vi "Skywater.vi"() -> ()   [LabVIEW 2018]
uses:
  Globals.vi
  <vilib>/Utility/file.llb/Write Delimited Spreadsheet (DBL).vi
panel:
  in  "current limit range (A)":dbl=3.2e-05 format="%#_6p"
  in  "RRAM Mode":u16(ring)=1 items=["1T1R", "1T4R", "1T8R"]
  in  "Addr hold time (s)":dbl=0.001 caption="Time Target (s)" format="%#_6p"
  in  "Initial address":i32
  in  "Stride":i32=8
  in  "Final address":i32=4096
  out "Current address":i32=4096
  in  "Mode":T1(tab)=enum."Target"
  in  "FORM outfile":path=path "C:/Users/RSG/Desktop/NI-Skywater-Test-Setup/eray/1T8R_form"
  out "FORM resistance (ohm)":dbl=10056.36151540716 format="%#_6p"
  out "FORM WL voltage (V)":dbl=1.2
  out "FORM BL voltage (V)":dbl=1.0
  out "formed?":bool=TRUE
  in  "SET target resistance (ohm)":dbl format="%#_6p"
  out "SET resistance (ohm)":dbl format="%#_6p"
  out "SET WL voltage (V)":dbl
  out "SET BL voltage (V)":dbl
  out "set?":bool
  in  "SET outfile":path=path "C:/Users/RSG/Desktop/NI-Skywater-Test-Setup/set.csv"
  in  "RESET target resistance (ohm)":dbl=50000.0 format="%#_6p"
  in  "RESET outfile":path=path "C:/Users/RSG/Desktop/NI-Skywater-Test-Setup/prereset.csv"
  out "reset?":bool=TRUE
  out "RESET SL voltage (V)":dbl=0.1
  out "RESET WL voltage (V)":dbl=0.1
  out "RESET resistance (ohm)":dbl=-27076590.237838075 format="%#_6p"
  in  "aperture time (s)":dbl=0.0005 format="%#_6p"
  in  "channel list":string="BL_SEL_0"
  in  "voltage level (V)":dbl=0.2 format="%#_6p"
  in  "settling time (s)":dbl=0.001 caption="Time Target (s)" format="%#_6p"
  out "currents (A)":dbl[][](array[numeric])=[[2.5991655032025314e-06], [2.6178851900457248e-06], [2.629369660501652e-06], [2.5730383329152406e-06], [2.541800573275067e-06], [2.630403262842684e-06], [2.5273875628528547e-06], [2.615186339488569e-06], [2.5948014044292527e-06], [2.4742144646418167e-06], [2.5204394582269958e-06], [2.4999971008154232e-06], [2.519922657056459e-06], [2.621330531182484e-06], [2.4824832833700937e-06], [2.4807606128016933e-06], [2.5330149533762534e-06], [2.6165644759432856e-06], [2.6238571146828077e-06], [2.569765258835313e-06], [2.5066006713275767e-06], [2.577459854040776e-06], [2.469792943516261e-06], [2.4861583139160038e-06], [2.607147210169401e-06], [2.5890591692012994e-06], [2.474673843460035e-06], [2.5888294797921905e-06], [2.6161050971250466e-06], [2.507749118373163e-06], [2.542030262684197e-06], [2.56959299177846e-06], [2.56224293068664e-06], [2.578608301086383e-06], [2.471630458789216e-06], [2.5237125323069446e-06], [2.5285934322507392e-06], [2.587336498632878e-06], [2.482311016313262e-06], [2.568214855323765e-06], [2.6001416831912863e-06], [2.592906466804041e-06], [2.4948865114625405e-06], [2.5907244174174017e-06], [2.5169366947379384e-06], [2.483287196301996e-06], [2.56482693653922e-06], [2.5010881255087116e-06], [2.5543186460720477e-06], [2.615817985363661e-06], [2.619837550023234e-06], [2.523310575841004e-06], [2.559946036595467e-06], [2.472491794073395e-06], [2.581594263404925e-06], [2.477085582255804e-06], [2.5706265941195135e-06], [2.4692187199934886e-06], [2.4722621046643074e-06], [2.48948881034823e-06], [2.573497711733479e-06], [2.603759291384898e-06], [2.5118261053850556e-06], [2.5823407539845498e-06], [2.503844398418165e-06], [2.6069749431125487e-06], [2.538872033308824e-06], [2.489718499757339e-06], [2.4820813269041528e-06], [2.5377235862631957e-06], [2.57389966819942e-06], [2.5408243932863126e-06], [2.531694239273856e-06], [2.5649417812437956e-06], [2.5744164693699567e-06], [2.5070600501458364e-06], [2.4714007693800864e-06], [2.5745887364268094e-06], [2.5535147331401244e-06], [2.5427193309115445e-06], [2.5436380885480013e-06], [2.568214855323765e-06], [2.6206988853074342e-06], [2.5368048286267393e-06], [2.5548354472425636e-06], [2.6078937007490262e-06], [2.56333395537997e-06], [2.6108222407152904e-06], [2.618861370034479e-06], [2.551504950810338e-06], [2.577804388154481e-06], [2.516190204158293e-06], [2.4707691235050155e-06], [2.631207175774628e-06], [2.567468364744098e-06], [2.481736792790448e-06], [2.624948139376138e-06], [2.6001991055435636e-06], [2.6293122381493748e-06], [2.6262688534785556e-06], [2.621387953534782e-06], [2.6042186702031576e-06], [2.6057116513624076e-06], [2.6274747228764197e-06], [2.5883126786216535e-06], [2.5067155160321314e-06], [2.6222492888189616e-06], [2.485641512745488e-06], [2.517855452374416e-06], [2.6282212134560864e-06], [2.6235700029214215e-06], [2.5512178390489516e-06], [2.56224293068664e-06], [2.4763965140284565e-06], [2.6070323654648468e-06], [2.5409966603431653e-06], [2.473295707005339e-06], [2.5963518079408215e-06], [2.4696780988116856e-06], [2.5257223146367313e-06], [2.497700206724229e-06], [2.5825704433937e-06], [2.5093569442370093e-06], [2.618000034750258e-06], [2.5005139019859395e-06], [2.553916689606086e-06], [2.5049354231114744e-06], [2.623971959387404e-06], [2.618000034750258e-06], [2.505969025452506e-06], [2.5621855083343838e-06], [2.5615538624593132e-06], [2.629139971092564e-06], [2.63137944283146e-06], [2.5304883698759716e-06], [2.482253593960964e-06], [2.5134913536011584e-06], [2.512974552430642e-06], [2.4726066387779705e-06], [2.5681574329714667e-06], [2.607262054873977e-06], [2.543810355604854e-06], [2.5335891768990678e-06], [2.575335227006434e-06], [2.625752052308061e-06], [2.5207265699883824e-06], [2.481564525733637e-06], [2.5329575310239765e-06], [2.482311016313262e-06], [2.599854571429879e-06], [2.5806180834161697e-06], [2.6027831113961435e-06], [2.625005561728436e-06], [2.5987061243842925e-06], [2.5584530554362175e-06], [2.544556846184479e-06], [2.5993951926116403e-06], [2.5287082769552935e-06], [2.6237996923305516e-06], [2.5749906928927503e-06], [2.509242099532476e-06], [2.532096195739776e-06], [2.573612556438034e-06], [2.5942271809064803e-06], [2.6215027982393368e-06], [2.470654278800461e-06], [2.6146695383180532e-06], [2.510447968930319e-06], [2.4926470397236026e-06], [2.5546057578334547e-06], [2.59313615621315e-06], [2.616162519477324e-06], [2.604850316078228e-06], [2.517453495908475e-06], [2.6008307514186338e-06], [2.589920504485479e-06], [2.5769430528702803e-06], [2.578608301086383e-06], [2.5006287466904938e-06], [2.5325555745580356e-06], [2.562013241277531e-06], [2.563276533027693e-06], [2.561496440107015e-06], [2.5335891768990678e-06], [2.6061710301806466e-06], [2.6077214336922154e-06], [2.5973854102818537e-06], [2.5887720574398924e-06], [2.535771226285707e-06], [2.6041612478508595e-06], [2.625177828785226e-06], [2.5608073718796465e-06], [2.6279341016946795e-06], [2.6260391640694467e-06], [2.6308052193086663e-06], [2.567640631800951e-06], [2.607836278396749e-06], [2.6220195994098734e-06], [2.6283360581606407e-06], [2.5542612237197704e-06], [2.6263836981831314e-06], [2.4892016985868226e-06], [2.603185067862126e-06], [2.5605202601182815e-06], [2.5732680223243495e-06], [2.5300864134099892e-06], [2.6169090100569907e-06], [2.4893739656436753e-06], [2.4796121657560857e-06], [2.5791825246091555e-06], [2.6038741360894526e-06], [2.5487486779009052e-06], [2.4730660175962303e-06], [2.497700206724229e-06], [2.5769430528702803e-06], [2.5582807883793648e-06], [2.5942846032587576e-06], [2.5919877091675636e-06], [2.545360759116402e-06], [2.5386997662519713e-06], [2.5909541068265106e-06], [2.5470260073325256e-06], [2.566032805937126e-06], [2.5914134856447708e-06], [2.583087244564216e-06], [2.5805032387116155e-06], [2.5981319008614785e-06], [2.4712859246755525e-06], [2.5709711282331555e-06], [2.5671812529827123e-06], [2.4912114809165884e-06], [2.5096440559984163e-06], [2.499824833758571e-06], [2.543867777957152e-06], [2.6064581419420536e-06], [2.623512580569123e-06], [2.4878809844843626e-06], [2.4827129727792026e-06], [2.5833743563255815e-06], [2.615358606545422e-06], [2.537321629797255e-06], [2.5223918182045266e-06], [2.630001306376764e-06], [2.574186779960827e-06], [2.5205543029315716e-06], [2.629943884024466e-06], [2.4911540585643323e-06], [2.6046780490213754e-06], [2.5598886142431898e-06], [2.592906466804041e-06], [2.4807031904493948e-06], [2.56959299177846e-06], [2.5762539846429117e-06], [2.5793547916660083e-06], [2.624488760557899e-06], [2.519635545295094e-06], [2.490063033871002e-06], [2.5528830872650543e-06], [2.5377810086154937e-06], [2.610477706601648e-06], [2.540135325058944e-06], [2.5798141704842676e-06], [2.475879712857919e-06], [2.584293113962059e-06], [2.625292673489801e-06], [2.6155882959545307e-06], [2.4764539363807334e-06], [2.6153011841931238e-06], [2.6170812771137803e-06], [2.554663180185711e-06], [2.544556846184479e-06], [2.54237479679784e-06], [2.601462397293725e-06], [2.580273549302486e-06], [2.4928193067804553e-06], [2.547944764969003e-06], [2.573497711733479e-06], [2.5141229994762497e-06], [2.56810001061919e-06], [2.6310923310700733e-06], [2.5039592431227196e-06], [2.5781489222681238e-06], [2.6303458404904065e-06], [2.6269004993536473e-06], [2.5631616883231175e-06], [2.5672960976872873e-06], [2.593767802088221e-06], [2.6223067111712596e-06], [2.475305489335126e-06], [2.620296928841452e-06], [2.5483467214349647e-06], [2.481909059847301e-06], [2.5135487759534145e-06], [2.5127448630214917e-06], [2.5707414388240677e-06], [2.5985338573274397e-06], [2.596926031463636e-06], [2.6220770217621507e-06], [2.5457627155823845e-06], [2.478176606949113e-06], [2.554433490776602e-06], [2.6308052193086663e-06], [2.6127171783405435e-06], [2.6221918664666842e-06], [2.473812508175855e-06], [2.6189187923867565e-06], [2.5029256407816874e-06], [2.6084679242718614e-06], [2.4769133151989516e-06], [2.6224789782280912e-06], [2.533991133365029e-06], [2.6215602205916137e-06], [2.5078065407254612e-06], [2.6166793206478403e-06], [2.5091846771801773e-06], [2.6206988853074342e-06], [2.554146379015195e-06], [2.6041038254986034e-06], [2.57522038230188e-06], [2.5267559169777634e-06], [2.599854571429879e-06], [2.6041612478508595e-06], [2.4777746504831306e-06], [2.613578513624744e-06], [2.5751055375973045e-06], [2.577746965802183e-06], [2.47369766347128e-06], [2.561726129516124e-06], [2.6300587287290415e-06], [2.5759668728815047e-06], [2.551906907276299e-06], [2.571545351755991e-06], [2.5317516616261127e-06], [2.6150140724317164e-06], [2.5413986168091058e-06], [2.617253544170633e-06], [2.5444420014799246e-06], [2.5085530313050864e-06], [2.516075359453738e-06], [2.4776598057785764e-06], [2.5530553543219066e-06], [2.607549166635384e-06], [2.606917520760292e-06], [2.608927303090079e-06], [2.6161050971250466e-06], [2.5607499495273696e-06], [2.5237699546592012e-06], [2.6057690737147057e-06], [2.625292673489801e-06], [2.563793334198188e-06], [2.4999971008154232e-06], [2.622134444114407e-06], [2.586360318644123e-06], [2.516821850033384e-06], [2.631034908717775e-06], [2.6286231699220273e-06], [2.5600034589477444e-06], [2.551906907276299e-06], [2.4902353009278548e-06], [2.4784062963582427e-06], [2.6220770217621507e-06], [2.5276746746142617e-06], [2.4739273528804097e-06], [2.6163922088864536e-06], [2.5186593653063185e-06], [2.5049354231114744e-06], [2.5821110645754197e-06], [2.6227086676372213e-06], [2.6302884181381504e-06], [2.6271876111150543e-06], [2.553399888435549e-06], [2.6008307514186338e-06], [2.615645718306829e-06], [2.614037892442962e-06], [2.4816219480858723e-06], [2.6233977358645687e-06], [2.5385849215474166e-06], [2.5449013802981635e-06], [2.606056185476071e-06], [2.6290251263879886e-06], [2.5384126544905643e-06], [2.6303458404904065e-06], [2.6101331724879637e-06], [2.622134444114407e-06], [2.623512580569123e-06], [2.6264411205353875e-06], [2.6242016487964916e-06], [2.5740145129039747e-06], [2.5626448871526016e-06], [2.597787366747815e-06], [2.600084260839009e-06], [2.4742144646418167e-06], [2.5307180592850805e-06], [2.6121429548177503e-06], [2.60525227254419e-06], [2.480530923392605e-06], [2.5884849456784855e-06], [2.6082382348627105e-06], [2.4721472599597527e-06], [2.5414560391613623e-06], [2.5475428085030415e-06], [2.61409531479526e-06], [2.510907347748578e-06], [2.4979873184856366e-06], [2.5218175946817123e-06], [2.5273875628528547e-06], [2.5907244174174017e-06], [2.6175406559320608e-06], [2.5682722776760214e-06], [2.561209328345608e-06], [2.514410111237636e-06], [2.4940251761782983e-06], [2.497298250258268e-06], [2.4703097446867977e-06], [2.5262391158072476e-06], [2.5704543270626608e-06], [2.561726129516124e-06], [2.591528330349325e-06], [2.4819664821995778e-06], [2.6217899100007645e-06], [2.5914134856447708e-06], [2.5849247598371503e-06], [2.546681473218862e-06], [2.532153618092074e-06], [2.503385019599905e-06], [2.5940549138496275e-06], [2.606917520760292e-06], [2.4925896173713464e-06], [2.56333395537997e-06], [2.483402041006571e-06], [2.573669978790332e-06], [2.6061710301806466e-06], [2.613061712454228e-06], [2.5511029943443973e-06], [2.615128917136292e-06], [2.5571897636860553e-06], [2.618976214739055e-06], [2.6184019912162406e-06], [2.6062284525329235e-06], [2.580388394007061e-06], [2.4821387492564098e-06], [2.5208414146929366e-06], [2.533474332194513e-06], [2.5848673374848734e-06], [2.513663620657969e-06], [2.4894313879959315e-06], [2.5806180834161697e-06], [2.5439252003094294e-06], [2.591011529178809e-06], [2.5729234882106656e-06], [2.4692187199934886e-06], [2.5856138280644982e-06], [2.5888869021444467e-06], [2.603529601975789e-06], [2.5286508546030166e-06], [2.4697355211639833e-06], [2.5208414146929366e-06], [2.4970111384968606e-06], [2.6300587287290415e-06], [2.6188039476822023e-06], [2.6230532017509264e-06], [2.5888869021444467e-06], [2.6261540087740225e-06], [2.5642527130164477e-06], [2.5934806903268135e-06], [2.6163922088864536e-06], [2.569765258835313e-06], [2.4956330020421652e-06], [2.5973854102818537e-06], [2.559084701311267e-06], [2.5985338573274397e-06], [2.543580666195745e-06], [2.609329259556041e-06], [2.5145823782944467e-06], [2.5898630821332227e-06], [2.5716601964605453e-06], [2.543810355604854e-06], [2.609501526612872e-06], [2.4861583139160038e-06], [2.6295993499107818e-06], [2.586130629235035e-06], [2.6282786358083426e-06], [2.4804160786880505e-06], [2.588714635087615e-06], [2.5631042659708406e-06], [2.6056542290101515e-06], [2.5608073718796465e-06], [2.4733531293576372e-06], [2.5163624712151456e-06], [2.5867622751101054e-06], [2.494197443235151e-06], [2.623455158216867e-06], [2.6243164935010463e-06], [2.5285934322507392e-06], [2.6139804700907053e-06], [2.6117409983517886e-06], [2.623627425273699e-06], [2.499193187883479e-06], [2.509758900702971e-06], [2.5946865597246985e-06], [2.5642527130164477e-06], [2.579871592836545e-06], [2.610994507772143e-06], [2.621330531182484e-06], [2.5015475043269713e-06], [2.549437746128253e-06], [2.5690761906079443e-06], [2.5115964159759052e-06], [2.601634664350536e-06], [2.5436380885480013e-06], [2.576770785813428e-06], [2.5669515635735822e-06], [2.610707396010757e-06]] format="%#_6p"
  out "resistances (ohm)":dbl[][](array[numeric])=[[76947.77410425474], [76397.5443844834], [76063.85781520062], [77729.11792316787], [78684.37913770057], [76033.96894507327], [79133.09495526867], [76476.38601504487], [77077.18966800529], [80833.73646793117], [79351.24144608104], [80000.09277401405], [79367.51528462446], [76297.13140745355], [80564.49013766978], [80620.43510684663], [78957.291481213], [76436.10613795364], [76223.66282097551], [77828.12041386435], [79789.33473039945], [77595.77697648825], [80978.44822378457], [80445.39998942205], [76712.20068428927], [77248.13800284763], [80818.73113442876], [77254.99171001959], [76449.52804831459], [79752.79446204922], [78677.26947861537], [77833.33805778188], [78056.61110611523], [77561.21777616974], [80918.24539902074], [79248.32857931664], [79095.35690835715], [77299.57046780655], [80570.08114037248], [77875.10440779955], [76918.88534109796], [77133.51891420734], [80163.96701057034], [77198.48497022802], [79461.67276202545], [80538.40904822903], [77977.97081383767], [79965.19513254687], [78298.76679933956], [76457.91913621822], [76340.61127119363], [79260.95262107845], [78126.64686712879], [80890.05612855962], [77471.50775591488], [80740.0444428191], [77802.04268387867], [80997.27998195616], [80897.5713467714], [80337.77824935233], [77715.2429893875], [76812.01586557689], [79623.3463659064], [77449.11266702513], [79877.16813646747], [76717.2697721497], [78775.14005278437], [80330.36667377982], [80577.53701787675], [78810.78974976172], [77703.10648507549], [78714.60952927927], [78998.48129265574], [77974.47936733118], [77687.50797688398], [79774.71460580529], [80925.7658563273], [77682.30986575887], [78323.41729004036], [78655.94820813417], [78627.53781697266], [77875.10440779955], [76315.5206884968], [78839.33274767021], [78282.92824724199], [76690.24237550671], [78023.38808809384], [76604.21949876058], [76369.06721693592], [78385.11147567305], [77585.40598310695], [79485.24704908121], [80946.45432361621], [76010.73828066008], [77897.74656870376], [80588.72342184256], [76191.98147188283], [76917.18667759122], [76065.51899700158], [76153.66558343609], [76295.46009407428], [76798.46638392998], [76754.46356293074], [76118.71515211025], [77270.41699865466], [79785.67919688753], [76270.39917706615], [80462.125762895], [79432.6774443679], [76097.09524298446], [76232.00439755531], [78393.93286562955], [78056.61110611523], [80762.51071547979], [76715.58000176151], [78709.2730664942], [80863.76385707618], [77031.16326081438], [80982.21387484965], [79185.26864215694], [80073.66114698889], [77442.2244750793], [79701.69427642414], [76394.1930272277], [79983.55851617441], [78311.09010484122], [79842.37763366071], [76220.32670146837], [76394.1930272277], [79809.44615382297], [78058.36046977539], [78077.60864648878], [76070.50297778103], [76005.76212786429], [79036.12693142025], [80571.94498039076], [79570.59399207946], [79586.9579365826], [80886.29904303963], [77876.84564516418], [76708.82166452083], [78622.21315332489], [78939.39626186188], [77659.79275345824], [76168.65416679313], [79342.20330804137], [80594.31778864305], [78959.08144940266], [80570.08114037248], [76927.37978417122], [77500.81319094071], [76840.82439459168], [76190.31476196565], [76961.376326223], [78172.23754605882], [78599.14794196747], [76940.9747961632], [79091.76468580679], [76225.33099024527], [77670.18364455507], [79705.34211795035], [78985.94071445541], [77711.77502988512], [77094.25044653013], [76292.11768697128], [80950.21699964552], [76491.50191601446], [79667.05642786868], [80235.98881539884], [78289.96681257729], [77126.6867421521], [76447.85005174582], [76779.84364994647], [79445.36029168073], [76898.5063295292], [77222.44742787292], [77611.33866626727], [77561.21777616974], [79979.88516475864], [78971.61349949948], [78063.60903125985], [78025.1359629013], [78079.35895145898], [78939.39626186188], [76740.9343761054], [76695.30856170646], [77000.50951556594], [77256.70532684345], [78871.46834336146], [76800.15980771327], [76185.31506970251], [78100.36873378685], [76105.40913907459], [76160.3264477098], [76022.35183817858], [77892.52028611161], [76691.93102987141], [76277.08047835079], [76093.77019313269], [78300.5270340909], [76150.33558819116], [80347.04464228216], [76828.95944246126], [78109.1261471843], [77722.17983704104], [79048.68345205841], [76426.04279758448], [80341.4845500267], [80657.77493837058], [77543.94971728789], [76808.62804696229], [78469.87886020826], [80871.27419040594], [80073.66114698889], [77611.33866626727], [78177.50143317819], [77092.544028814], [77160.8597111101], [78574.32361353292], [78780.48545112979], [77191.64128498087], [78522.95164015933], [77941.3262126862], [77177.95755401725], [77426.73052212037], [77504.26234684956], [76978.3858678171], [80929.52660921152], [77791.61648440825], [77906.45859836639], [80282.22474569452], [79692.57613324518], [80005.60571249838], [78620.438425699], [76732.48105606691], [76233.67293196425], [80389.69759699013], [80557.03667432634], [77418.1254490993], [76471.34870891616], [78823.2747678823], [79289.82268201408], [76045.5896029691], [77694.43987395643], [79347.62594378021], [76047.24998692764], [80284.07529129743], [76784.92168164262], [78128.39937144233], [77133.51891420734], [80622.30127731193], [77833.33805778188], [77632.0972979384], [77538.7707988864], [76205.31777681728], [79376.55919065725], [80319.25187415196], [78342.79642404748], [78809.00649859918], [76614.32981948828], [78735.96261858962], [77524.9637311889], [80779.36862657157], [77390.60206424259], [76181.98230604896], [76464.63333290462], [80760.63804856967], [76473.02773722571], [76421.01212101744], [78288.20705258728], [78599.14794196747], [78666.60739868216], [76879.83505279876], [77511.16157977325], [80230.44408232922], [78494.63722673482], [77715.2429893875], [79550.60275160152], [77878.58696039583], [76014.05607786459], [79873.50455056826], [77575.03776160852], [76035.62882161216], [76135.35421277293], [78028.63194746207], [77902.97355266781], [77107.90450825308], [76268.72903462521], [80798.10789484435], [76327.2275743302], [78482.25609087477], [80583.12983164056], [79568.77619139815], [79594.23296144229], [77798.56697353658], [76966.47839936077], [77014.13038987458], [76275.41004329127], [78561.91732867247], [80704.49839578637], [78295.24656725189], [76022.35183817858], [76548.66039768957], [76272.06939265406], [80846.87070625107], [76367.3927505517], [79906.4889269096], [76673.35992096926], [80745.65983910322], [76263.71904614173], [78926.87443401145], [76290.44659323734], [79750.96832714368], [76432.75139671445], [79707.166163935], [76315.5206884968], [78304.04774103599], [76801.85330617774], [77663.25607489505], [79152.87687906901], [76927.37978417122], [76800.15980771327], [80717.59066588354], [76523.43289378445], [77666.7197052473], [77587.13428948249], [80850.62412976728], [78072.35820238807], [76043.92929151384], [77640.75000556115], [78372.76486447697], [77774.24569371453], [78996.68953768653], [76481.42398485025], [78696.82413344242], [76415.98210668462], [78602.69555512523], [79727.23618122957], [79488.87510405164], [80721.33209472327], [78337.51025469643], [76700.37541729935], [76718.95961697752], [76659.8593081206], [76449.52804831459], [78102.1200593652], [79246.52547304262], [76752.77215370664], [76181.98230604896], [78009.40790828169], [80000.09277401405], [76273.73968139438], [77328.74594397128], [79465.29866519838], [76015.71508508385], [76085.45883962995], [78124.8944414346], [78372.76486447697], [80313.69562767043], [80697.01900526922], [76275.41004329127], [79124.10644005095], [80843.11763121853], [76441.13880201499], [79407.3238941845], [79842.37763366071], [77456.0020844364], [76257.04008527128], [76037.28877062463], [76127.0337732425], [78326.94005580875], [76898.5063295292], [76462.95467318292], [76509.98502286019], [80592.45291341183], [76237.01021991158], [78784.04945306627], [78588.5070236269], [76744.31622565507], [76073.82599449687], [78789.39606064095], [76035.62882161216], [76624.44280931505], [76273.73968139438], [76233.67293196425], [76148.67069977603], [76213.6553384622], [77699.63960862141], [78044.36775562119], [76988.59520222442], [76920.584079634], [80833.73646793117], [79028.95356762869], [76565.48797650091], [76767.99752090329], [80627.90030710901], [77265.27455139464], [76680.11201075249], [80901.32947956186], [78695.04603589234], [78507.02226963628], [76508.30437132104], [79652.48107594704], [80064.45770158942], [79307.877152488], [79133.09495526867], [77198.48497022802], [76407.60022074365], [77873.3632482986], [78088.11165356342], [79541.51914444719], [80191.65239801972], [80086.54952579903], [80961.5071268552], [79169.06944736741], [77807.2568317315], [78072.35820238807], [77174.53737927727], [80581.26547412327], [76283.76295030508], [77177.95755401725], [77371.69108651347], [78533.57481224822], [78984.14952829597], [79891.82584146177], [77099.37015296108], [76718.95961697752], [80237.83723006818], [78023.38808809384], [80534.68455672852], [77710.04116619621], [76740.9343761054], [76538.56740036841], [78397.4619775779], [76478.0652645648], [78210.85585440107], [76365.71835759388], [76382.46559196227], [76739.243563098], [77507.71180977988], [80575.6729191369], [79338.58862928986], [78942.97465676656], [77373.40988439428], [79565.14083919016], [80339.63135694458], [77500.81319094071], [78618.66377819328], [77189.93055325681], [77732.58743076329], [80997.27998195616], [77351.07146673683], [77253.27816921414], [76818.79239944968], [79093.56075629462], [80980.33100554033], [79338.58862928986], [80095.7580511215], [76043.92929151384], [76370.74175675194], [76247.0238371441], [77253.27816921414], [76156.99586992874], [77995.43273748977], [77116.44075313988], [76441.13880201499], [77828.12041386435], [80139.98846638945], [77000.50951556594], [78152.94268982994], [76966.47839936077], [78629.3128651296], [76648.05017134121], [79536.06997582359], [77224.15960123409], [77770.77246646587], [78622.21315332489], [76642.99022641295], [80445.39998942205], [76057.21381349814], [77335.6139628411], [76095.4326817365], [80631.6334257052], [77258.4190196889], [78030.38005722524], [76756.1550467028], [78100.36873378685], [80861.88649169667], [79479.80558755531], [77316.72984580194], [80186.11379080953], [76235.34153941392], [76210.32009488465], [79095.35690835715], [76511.66574823721], [76577.27168437281], [76230.33593618417], [80025.82632252465], [79688.9294601091], [77080.60121960181], [77995.43273748977], [77523.2381934567], [76599.16533897728], [76297.13140745355], [79950.51049562579], [78448.66983072381], [77848.99518790533], [79630.62804510655], [76874.7444599134], [78627.53781697266], [77616.52728333947], [77913.42962528282], [76607.5893091682]] format="%#_6p"
  in  "READ outfile":path=path "C:/Users/RSG/Desktop/NI-Skywater-Test-Setup/eray/initial_read.csv"
  in  "Sweep outfile":path=path "C:/Users/RSG/Desktop/NI-Skywater-Test-Setup/resist_sweep2.csv"
  in  "Algorithm":u16(ring)=2 items=["Ping-Pong", "ISPP", "Our Algorithm (opt)", "Our Algorithm (3-level)"]
  in  "Upper resistance (ohm)":dbl=81000.0 format="%#_6p"
  in  "Lower resistance (ohm)":dbl=76000.0 format="%#_6p"
  in  "Target outfile":path=path "C:/Users/RSG/Desktop/NI-Skywater-Test-Setup/eray/Lv8/Lv5.csv"
  in  "Perform retention test":bool
  in  "CB type":u16(ring)=2 items=["1 bit/cell"=1, "2 bit/cell"=2, "3 bit/cell"=3]
  in  "Read Ranges (multi-bit)":dbl[](array[numeric])=[0.0, 3875.0, 4750.0, 6050.0, 8300.0, 12200.0, 21100.0, 68000.0, 10000000000.0] format="%#_6p"
  in  "Write Targets (multi-bit)":dbl[][](array[numeric])=[[0.0, 3800.0], [3950.0, 4646.0], [4872.0, 5917.0], [6289.0, 7961.0], [8649.0, 11570.0], [13084.0, 18930.0], [23350.0, 48118.0], [92745.0, 10000000000.0]] format="%#_6p"
  in  "Read Ranges (1b)":dbl[](array[numeric])=[0.0, 7000.0, 1000000000.0] format="%#_6p"
  in  "Write Targets (1b)":dbl[][](array[numeric])=[[0.0, 6000.0], [15000.0, 30000.0]] format="%#_6p"
  in  "CB size":i32=4
  out "Checkerboard":T2(plugin-control)
  out "Confusion Matrix":i32[][](array[numeric])
  out "BER":dbl=nan
  # "Checkerboard Write"
  # "Checkerboard Read"
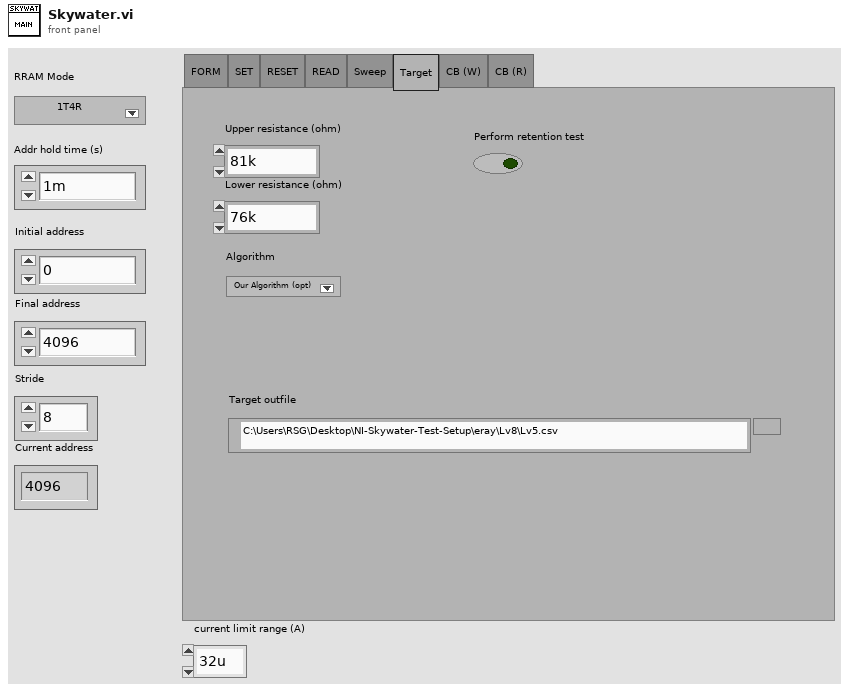
[diagram p1: front panel]
types:
  T1 = enum32{"FORM", "SET", "RESET", "READ", "Sweep", "Target", "CB (W)", "CB (R)"}
  T2 = typedef "IMAQ Image.ctl" = refnum<image>
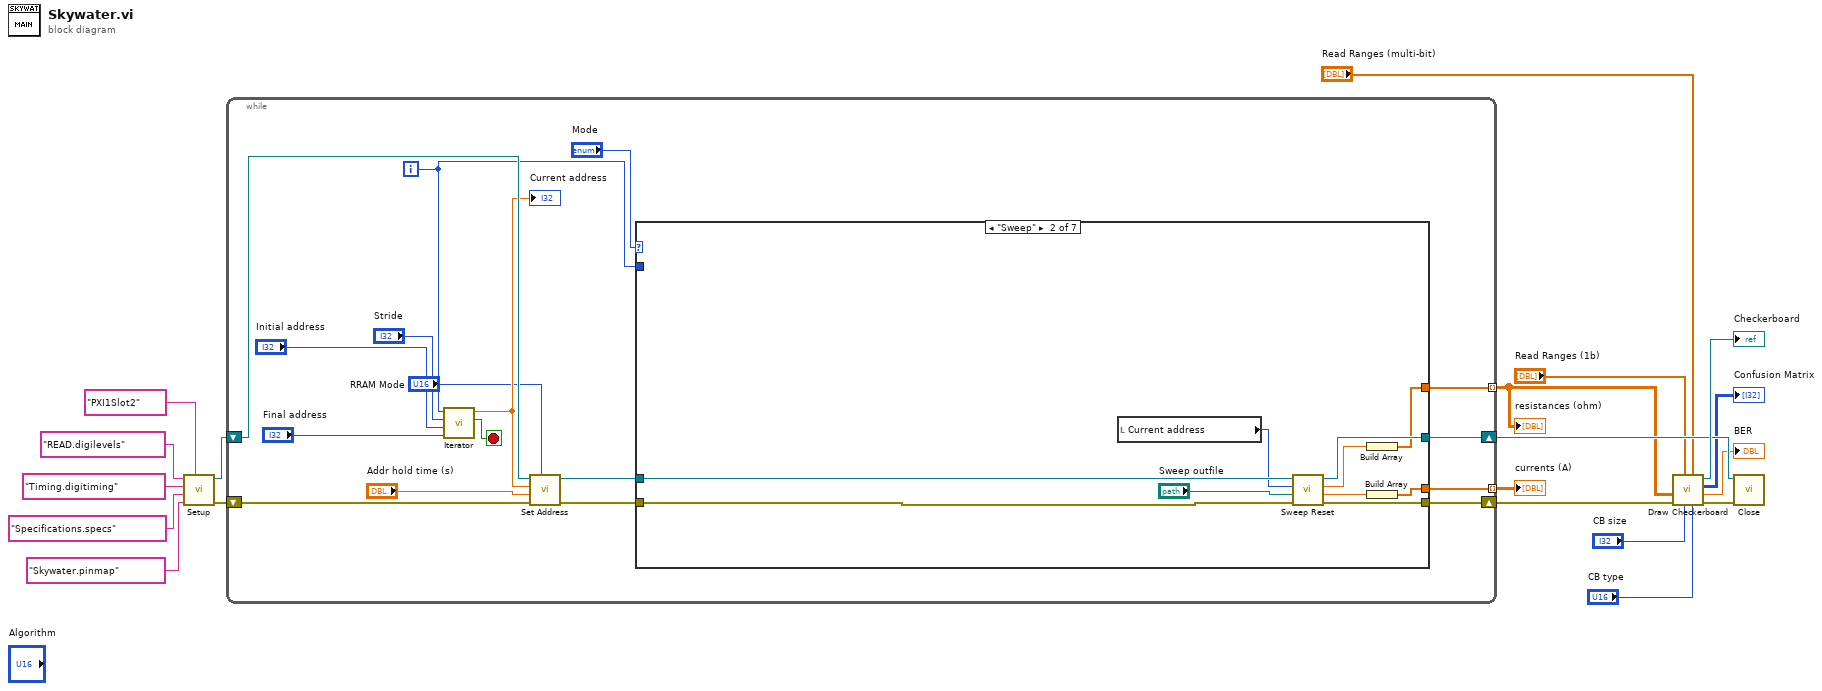
[diagram p0: block diagram]
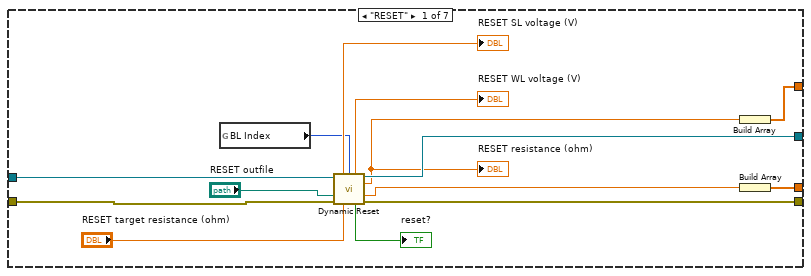
[diagram p2: hidden frame]
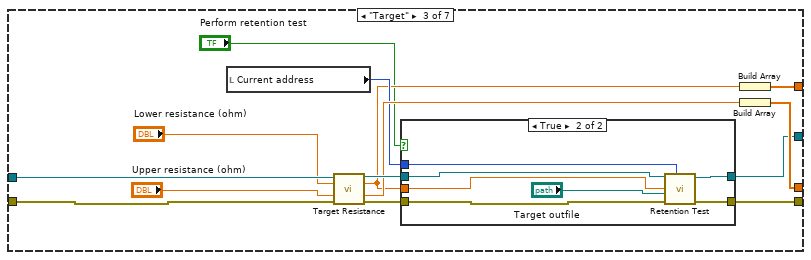
[diagram p3: hidden frame]
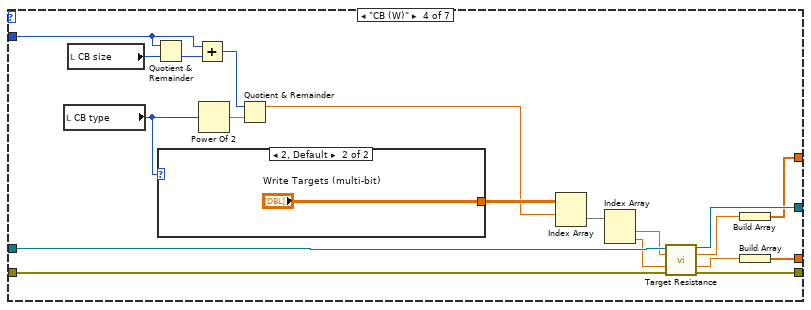
[diagram p5: hidden frame]
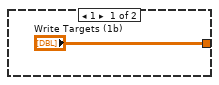
[diagram p6: hidden frame]
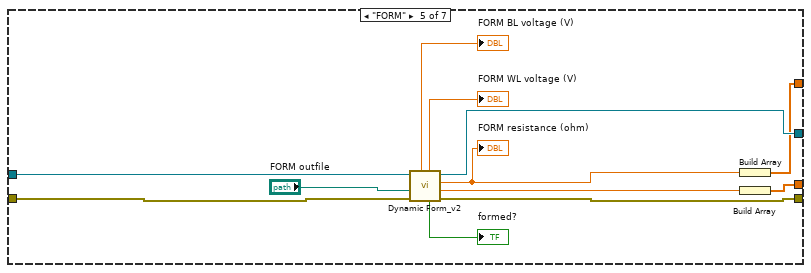
[diagram p7: hidden frame]
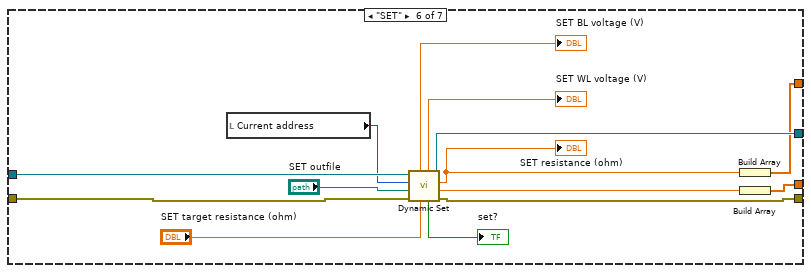
[diagram p8: hidden frame]
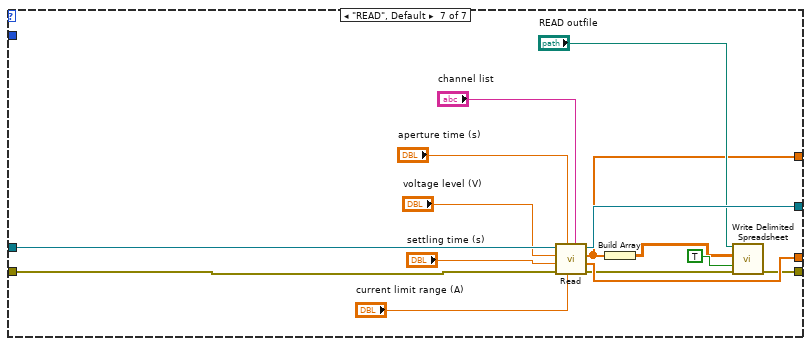
[diagram p9: hidden frame]
diagram:
  n1 = call "Setup.vi"("levels file path"="READ.digilevels" ("string"), "timing file path"="Timing.digitiming" ("name or relative path"), "specifications file path"="Specifications.specs" ("name or relative path"), "pin map file path"="Skywater.pinmap" ("file name"), "resource name"="PXI1Slot2" ("name or relative path")) -> ("instrument handle out"=w13:refnum<k15>, "error out"=w12:errorcluster)  [unwired: 4 in]
  n2 = while {
    tunnel: [w33] -> w8 mode=indexing
    tunnel: [w34] -> w11 mode=indexing
    shift-right: [w28] -> w7
    shift-left: w12 -> [w36]
    shift-right: [w29] -> w10
    shift-left: w13 -> [w23]
    i -> [w22]
    stop <- w27 stop-if-true
    n3 = call "Iterator.vi"("Final Value"="Final address", "Initial Value"="Initial address", "Step"="Stride", "i"=w22) -> ("End Loop"=w27:bool, "Current Value"=w21:dbl)  [unwired: 6 in]
    "Current address" <- w21
    n4 = call "Set Address.vi"("RRAM Mode"="RRAM Mode", "error in (no error)"=w36, "hold time (s)"="Addr hold time (s)", "address"=w21, "instrument handle"=w23) -> ("error out"=w30:errorcluster, "instrument handle out"=w32:refnum<k15>)  [unwired: 5 in]
    n5 = case shown="\"Sweep\"" "Mode" {
      tunnel: w32 -> [w45 w60 w73 w102 w115 w129 w145]
      tunnel: w30 -> [w44 w59 w74 w93 w116 w130 w144]
      tunnel: [w46 w57 w62 w101 w114 w128 w143] -> w29
      tunnel: [w48 w58 w68 w92 w113 w127 w134] -> w28
      tunnel: [w49 w52 w67 w91 w111 w125 w142] -> w34
      tunnel: [w50 w53 w66 w90 w112 w126 w133] -> w33
      tunnel: w22 -> [_ _ _ w85 _ _ _]
      frame "RESET" {
        n6 = global read "Globals.vi" "BL Index"() -> (w37:i32)
        n7 = call "Dynamic Reset.vi"("instrument handle"=w45, "index"=w37, "RESET outfile"="RESET outfile", "error in (no error)"=w44, "target resistance (ohm)"="RESET target resistance (ohm)") -> ("SL voltage (V)"=→"RESET SL voltage (V)":dbl, "WL voltage (V)"=→"RESET WL voltage (V)":dbl, "instrument handle out"=w46:refnum<k15>, "final resistance (ohm)"=w42:dbl, "final current (A)"=w47:dbl, "reset?"=→"reset?":bool, "error out"=w48:errorcluster)  [unwired: 4 in]
        "RESET resistance (ohm)" <- w42
        n8 = Build Array(w42) -> (w50:dbl[])
        n9 = Build Array(w47) -> (w49:dbl[])
      }
      frame "Sweep" {
        n10 = local read "Current address"() -> (w51:i32)
        n11 = call "Sweep Reset.vi"("error in (no error)"=w59, "Sweep outfile"="Sweep outfile", "addr"=w51, "instrument handle"=w60) -> ("error out"=w58:errorcluster, "final current (A)"=w54:dbl, "final resistance (ohm)"=w55:dbl, "instrument handle out"=w57:refnum<k15>)  [unwired: 4 in]
        n12 = Build Array(w55) -> (w53:dbl[])
        n13 = Build Array(w54) -> (w52:dbl[])
      }
      frame "Target" {
        n14 = local read "Current address"() -> (w64:i32)
        n15 = call "Target Resistance.vi"("instrument handle"=w73, "Lower resistance (ohm)"="Lower resistance (ohm)", "Upper resistance (ohm)"="Upper resistance (ohm)", "error in (no error)"=w74) -> ("instrument handle out"=w70:refnum<k15>, "final resistance (ohm)"=w63:dbl, "final current (A)"=w65:dbl, "error out"=w69:errorcluster)  [unwired: 5 in, 3 out]
        n16 = case shown="True" "Perform retention test" {
          tunnel: w70 -> [w76 w83]
          tunnel: w69 -> [w75 w82]
          tunnel: [w75 w81] -> w68
          tunnel: w64 -> [_ w77]
          tunnel: w63 -> [_ w78]
          tunnel: [w76 w80] -> w62
          frame False {
          }
          frame True {
            n17 = call "Retention Test.vi"("Current address"=w77, "error in (no error)"=w82, "target outfile"="Target outfile", "final resistance (ohm)"=w78, "IVI Refnum in"=w83) -> ("error out"=w81:errorcluster, "IVI Refnum out"=w80:refnum<k15>)  [unwired: 5 in]
          }
        }
        n18 = Build Array(w63) -> (w66:dbl[])
        n19 = Build Array(w65) -> (w67:dbl[])
      }
      frame "CB (W)" {
        n20 = local read "CB type"() -> (w98:u16)
        n21 = local read "CB size"() -> (w86:i32)
        n22 = Quotient & Remainder(x=w85, y=w86) -> (floor(x/y)=w84:i32)  [unwired: 1 out]
        n23 = case shown="2, Default" w98 {
          tunnel: ["Write Targets (1b)" "Write Targets (multi-bit)"] -> w100
          frame 1 {
          }
          frame 2, Default {
          }
        }
        n24 = Add(x=w85, y=w84) -> (x+y=w87:i32)
        n25 = Power Of 2(x=w98) -> (2^x=w99:dbl)
        n26 = Quotient & Remainder(x=w87, y=w99) -> (x-y*floor(x/y)=w97:dbl)  [unwired: 1 out]
        n27 = Index Array(array=w100, index (row)=w97) -> (element=w96:dbl[])  [unwired: 1 in]
        n28 = Index Array(array=w96) -> (element #1=w95:dbl, element #2=w94:dbl)  [unwired: 2 in]
        n29 = call "Target Resistance.vi"("instrument handle"=w102, "Lower resistance (ohm)"=w95, "Upper resistance (ohm)"=w94, "error in (no error)"=w93) -> ("instrument handle out"=w101:refnum<k15>, "final resistance (ohm)"=w89:dbl, "final current (A)"=w88:dbl, "error out"=w92:errorcluster)  [unwired: 5 in, 3 out]
        n30 = Build Array(w89) -> (w90:dbl[])
        n31 = Build Array(w88) -> (w91:dbl[])
      }
      frame "FORM" {
        n32 = call "Dynamic Form_v2.vi"("error in (no error)"=w116, "form outfile"="FORM outfile", "instrument handle"=w115) -> ("error out"=w113:errorcluster, "final current (A)"=w110:dbl, "final resistance (ohm)"=w109:dbl, "instrument handle out"=w114:refnum<k15>, "formed?"=→"formed?":bool, "WL voltage (V)"=→"FORM WL voltage (V)":dbl, "BL voltage (V)"=→"FORM BL voltage (V)":dbl)  [unwired: 2 in]
        "FORM resistance (ohm)" <- w109
        n33 = Build Array(w109) -> (w112:dbl[])
        n34 = Build Array(w110) -> (w111:dbl[])
      }
      frame "SET" {
        n35 = local read "Current address"() -> (w122:i32)
        n36 = call "Dynamic Set.vi"("target resistance (ohm)"="SET target resistance (ohm)", "error in (no error)"=w130, "SET outfile"="SET outfile", "addr"=w122, "instrument handle"=w129) -> ("error out"=w127:errorcluster, "final current (A)"=w124:dbl, "final resistance (ohm)"=w123:dbl, "instrument handle out"=w128:refnum<k15>, "SET?"=→"set?":bool, "WL voltage (V)"=→"SET WL voltage (V)":dbl, "BL voltage (V)"=→"SET BL voltage (V)":dbl)
        "SET resistance (ohm)" <- w123
        n37 = Build Array(w123) -> (w126:dbl[])
        n38 = Build Array(w124) -> (w125:dbl[])
      }
      frame "READ", Default {
        n39 = call "Read.vi"("channel list"="channel list", "current limit range (A)"="current limit range (A)", "aperture time (s)"="aperture time (s)", "error in (no error)"=w144, "settling time (s)"="settling time (s)", "voltage level (V)"="voltage level (V)", "instrument handle"=w145) -> ("error out"=w135:errorcluster, "currents (A)"=w142:dbl[], "resistances (ohm)"=w133:dbl[], "instrument handle out"=w143:refnum<k15>)  [unwired: 1 in]
        n40 = Build Array(w133) -> (w132:dbl[][])
        n41 = call-poly <vilib>:"Write Delimited Spreadsheet.vi"("file path (dialog if empty)"="READ outfile", "2D data"=w132, "append to file? (new file:F)"=TRUE, "error in (no error)"=w135) -> ("error out"=w134:errorcluster)  [unwired: 10 in, 1 out]
      }
    }
  }
  "resistances (ohm)" <- w8
  "currents (A)" <- w11
  n42 = call "Draw Checkerboard.vi"("CB type"="CB type", "Resistance Read Ranges (multi-bit)"="Read Ranges (multi-bit)", "CB size"="CB size", "Resistance Read Ranges (1b)"="Read Ranges (1b)", "error in (no error)"=w7, "Resistances (ohm)"=w8) -> ("error out"=w6:errorcluster, "BER"=→"BER":dbl, "Confusion Matrix"=→"Confusion Matrix":i32[][], "Checkerboard"=→"Checkerboard":T2)  [unwired: 2 in]
  n43 = call "Close.vi"("error in (no error)"=w6, "instrument handle"=w10) -> ()  [unwired: 10 in]
